vi "Set Report Tab Width.vi"(0 "report in":refnum<class "NI_report.lvclass">, 5 "width (.25)":dbl=0.25 format="%.2f", 9 "measurement system (US)":u16(ring)=1 items=["US", "Metric"], 11 "error in (no error)":errorcluster) -> (4 "report out":refnum<class "NI_report.lvclass">, 15 "error out":errorcluster)   [LabVIEW 2020, in "NI_report.lvclass"]
doc: "LabVIEW no longer supports this VI.\n\nSets the tab width in the report. You cannot use this VI with HTML reports.\n\nTo place a tab in the text, insert the token <tab> in the text string. Alternatively, you can use the Concatenate Strings function and insert a tab constant to build the text string."
uses:
  NI_report.lvclass
  NI_ReportGenerationCore.lvlib
panel:
  # "LabVIEW no longer supports this VI."
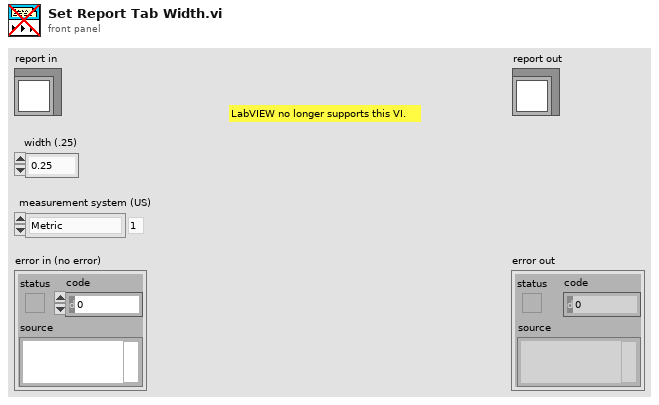
[diagram p1: front panel]
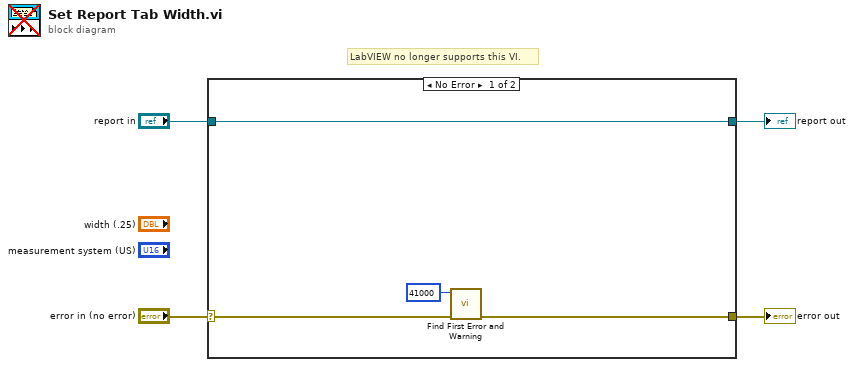
[diagram p0: block diagram]
diagram:
  # "LabVIEW no longer supports this VI."
  n1 = case shown="No Error" "error in (no error)" {
    selector: "error in (no error)" -> [w6 w10]
    tunnel: [w5 w10] -> w3
    tunnel: [w8 w9] -> w1
    tunnel: "report in" -> [w8 w9]
    frame No Error {
      n2 = call "Find First Error and Warning.vi"("error in (no error)"=w6, "error code"=41000) -> ("error out"=w5:errorcluster)  [unwired: 1 in, 4 out]
    }
    frame Error {
    }
  }
  "error out" <- w3
  "report out" <- w1
